vi "Init Msg.vi"(9 "Name Specs":refnum<class "Name Specs.lvclass">, 10 "Project Stuff":refnum<class "Project Stuff.lvclass">) -> (2 "Type":refnum<class "Type.lvclass">)   [LabVIEW 2020, in "_Rescript.lvlib" / "Msg.lvlib"]
uses:
  Msg.lvlib
  Type/Type.lvclass
  _Shared/Project Stuff/Project Stuff.lvclass
  _Shared/Name Specs/Name Specs.lvclass
  Msg/Msg.lvclass/Msg.ctl
  Msg/Msg.lvclass
  C:/git/jettl/src/jettl Tools/_Rescript/Type/Type.lvclass
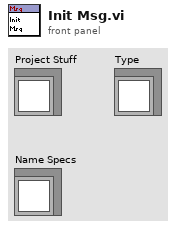
[diagram p1: front panel]
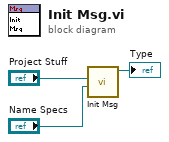
[diagram p0: block diagram]
diagram:
  n1 = call "Init Msg.vi"("Name Specs"="Name Specs", "Project Stuff"="Project Stuff") -> ("Msg out"=→"Type":refnum<class "Msg.lvclass">)  [unwired: 9 in]
